vi "Succeed.vi"(11 "Node In":refnum<class "bt_Node.lvclass">) -> (3 "Node":refnum<class "bt_Node.lvclass">)   [LabVIEW 2021, in "BT.lvlib"]
uses:
  BT.lvlib
  Support/Nodes/Decorators/Succeed/bt_Succeed.lvclass
  C:/Users/Tim/Documents/GitHub/LV_Behaviour_Tree/Source/Support/Nodes/Decorators/abs_Decorator/abs_Decorator.lvclass
  C:/Users/Tim/Documents/GitHub/LV_Behaviour_Tree/Source/Support/Nodes/abs_Node/bt_Node.lvclass
  C:/Users/Tim/Documents/GitHub/LV_Behaviour_Tree/Source/Support/Nodes/Decorators/Succeed/bt_Succeed.lvclass
  Support/Nodes/abs_Node/bt_Node.lvclass
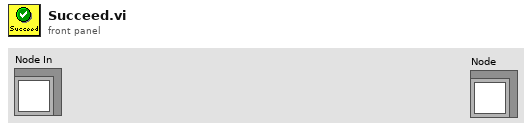
[diagram p1: front panel]
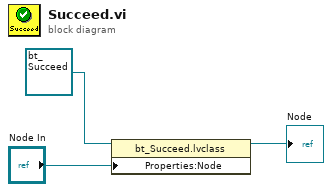
[diagram p0: block diagram]
diagram:
  n1 = property class="bt_Succeed.lvclass"(reference=refnum<class "bt_Succeed.lvclass"> refnum ("BT.lvlib:Succeed.lvclass"), "Properties:Node"="Node In") -> (reference out=→"Node":refnum<class "bt_Succeed.lvclass">)  [unwired: 1 in, 1 out]
